vi "lab6-Thermoister.vi"() -> ()   [LabVIEW 2016]
uses:
  <vilib>/DAQmx/read.llb/DAQmx Read (Analog DBL 1Chan 1Samp).vi
  <vilib>/DAQmx/write.llb/DAQmx Write (Analog DBL 1Chan 1Samp).vi
  <vilib>/DAQmx/miscellaneous.llb/DAQmx Fill In Error Info.vi
panel:
  in  "task/channels in 2":refnum<k21>
  out "LED Voltage":i32
  out "Heater On":bool
  in  "Slide":dbl(slide) scale=15.0..45.0 scale format="%#.3g"
  out "Thermometer":dbl(slide) min=-25.0 max=125.0 scale=15.0..45.0
  out "T":dbl
  in  "stop":bool
  out "Waveform Chart":dbl(graph)
  out "Vo":dbl format="%0.2f"
  in  "task/channels in":refnum<k21>
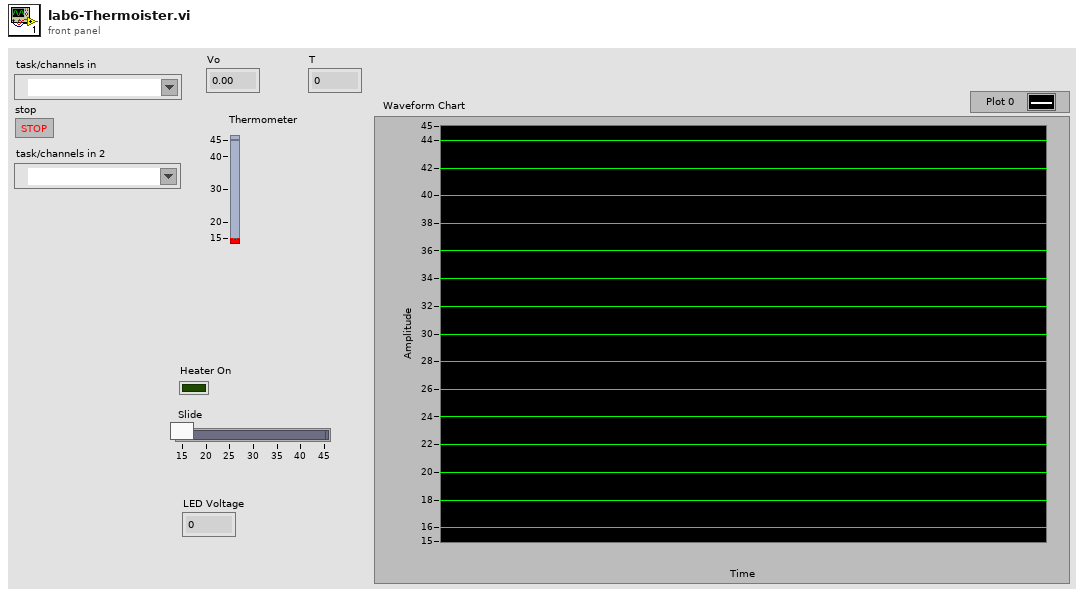
[diagram p1: front panel]
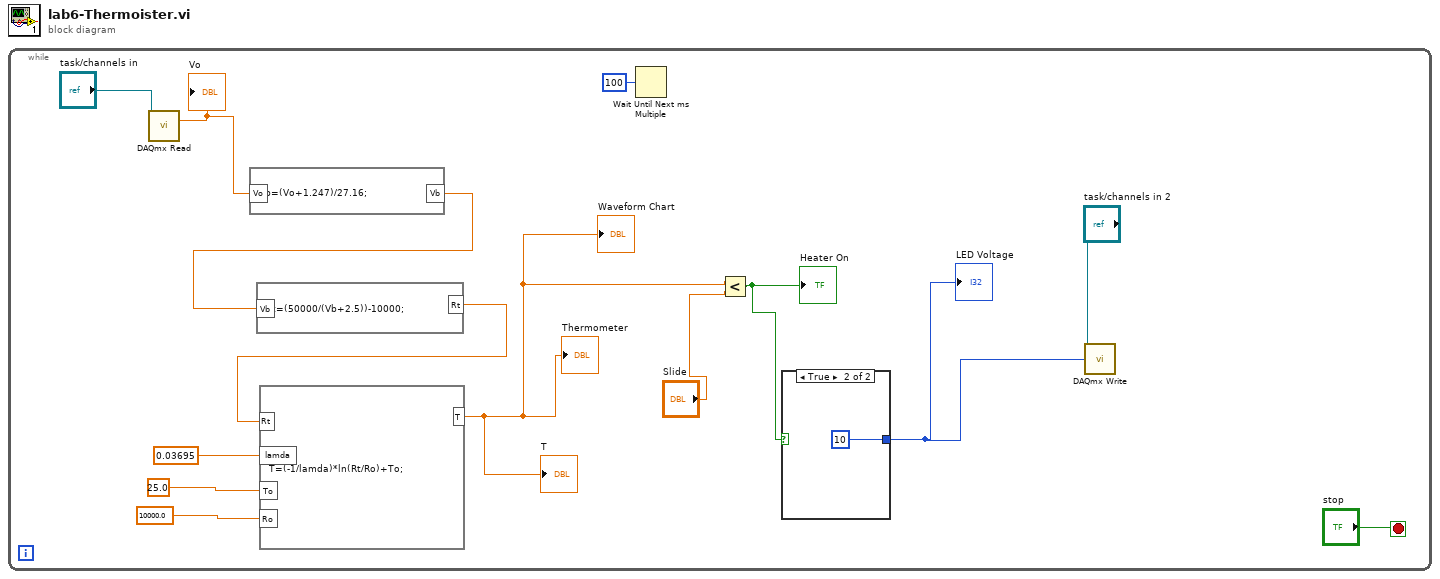
[diagram p0: block diagram]
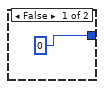
[diagram p2: hidden frame]
diagram:
  n1 = while {
    stop <- "stop" stop-if-true
    n2 = call-poly <vilib>:"DAQmx Read.vi"("task/channels in"="task/channels in") -> ("data"=w11:dbl)  [unwired: 12 in, 2 out]
    "Vo" <- w11
    n3 = formula code="Vb=(Vo+1.247)/27.16;"("Vo"=w11) -> ("Vb"=w7:dbl)
    n4 = formula code="Rt=(50000/(Vb+2.5))-10000;"("Vb"=w7) -> ("Rt"=w10:dbl)
    n5 = formula code="T=(-1/lamda)*ln(Rt/Ro)+To;"("Rt"=w10, "lamda"=0.03695 ("input variable"), "To"=25.0 ("input variable"), "Ro"=10000.0 ("input variable")) -> ("T"=w2:dbl)
    "Waveform Chart" <- w2
    "T" <- w2
    "Thermometer" <- w2
    n6 = Wait Until Next ms Multiple(millisecond multiple=u32 100) -> ()  [unwired: 1 out]
    n7 = Less?(x=w2, y="Slide") -> (x < y?=w3:bool)
    "Heater On" <- w3
    n8 = case shown="True" w3 {
      tunnel: [0 10] -> w9
      frame False {
      }
      frame True {
      }
    }
    "LED Voltage" <- w9
    n9 = call-poly <vilib>:"DAQmx Write.vi"("task/channels in"="task/channels in 2", "data"=w9) -> ()  [unwired: 11 in, 3 out]
  }
